vi "RSZVB Configure ZVAX Path.vi"(5 "Internal Combiner (Off)":bool, 6 "Pulse Modulator (Off)":bool, 7 "Harmonic Filter (Off)":bool, 8 "error in (no error)":errorcluster {"code" format="%.0x"}, 9 "Path (1)":i32=1, 10 "Channel (1)":i32=1, 11 "VISA session":refnum<visa-resource-name>) -> (0 "error out":errorcluster {"code" format="%.0x"}, 3 "dup VISA session":refnum<visa-resource-name>)   [LabVIEW 2011]
doc: "This VI configures the different signal paths in the Extension Unit R&S ZVAX24.\n\nRemote-control command(s):\n[SENSe<Ch>:]EUNit:COMBiner[:STATe] \n[SENSe<Ch>:]EUNit:HFILter<Path>[:STATe] \n[SENSe<Ch>:]EUNit:PMODulator<Path>[:STATe]"
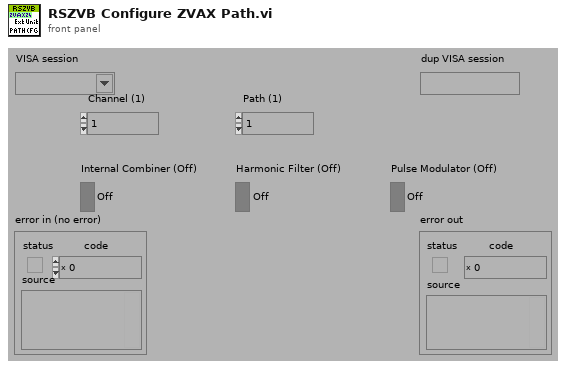
[diagram p1: front panel]
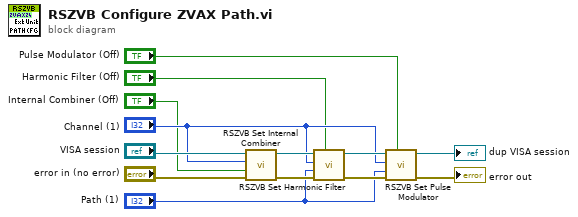
[diagram p0: block diagram]
diagram:
  n1 = call "RSZVB Set Internal Combiner.vi"("error in (no error)"="error in (no error)", "Internal Combiner (Off)"="Internal Combiner (Off)", "Channel (1)"="Channel (1)", "VISA session"="VISA session") -> ("error out"=w11:errorcluster, "dup VISA session"=w10:refnum<visa-resource-name>)  [unwired: 6 in]
  n2 = call "RSZVB Set Harmonic Filter.vi"("Harmonic Filter (Off)"="Harmonic Filter (Off)", "error in (no error)"=w11, "Path (1)"="Path (1)", "Channel (1)"="Channel (1)", "VISA session"=w10) -> ("error out"=w8:errorcluster, "dup VISA session"=w9:refnum<visa-resource-name>)  [unwired: 5 in]
  n3 = call "RSZVB Set Pulse Modulator.vi"("Pulse Modulator (Off)"="Pulse Modulator (Off)", "error in (no error)"=w8, "Path (1)"="Path (1)", "Channel (1)"="Channel (1)", "VISA session"=w9) -> ("error out"=→"error out":errorcluster, "dup VISA session"=→"dup VISA session":refnum<visa-resource-name>)  [unwired: 5 in]
